vi "Master VI.vi"() -> ()   [LabVIEW 2010]
panel:
  in  "GO Button":bool
  in  "Exec File":path
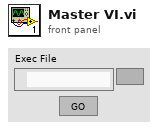
[diagram p1: front panel]
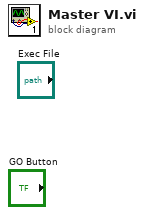
[diagram p0: block diagram]
diagram:
